vi "svl_Peak Level (1 Ch).vi"(8 "error in (no error)":errorcluster, 9 "processing state":T1(ring), 11 "scaled signal":waveform(dbl)={"t0"=timestamp(0 s since 1904-01-01), "dt"=0.0, "Y"=[]}) -> (0 "error out":errorcluster, 3 "peak level":dbl format="%.2f")   [LabVIEW 2017]
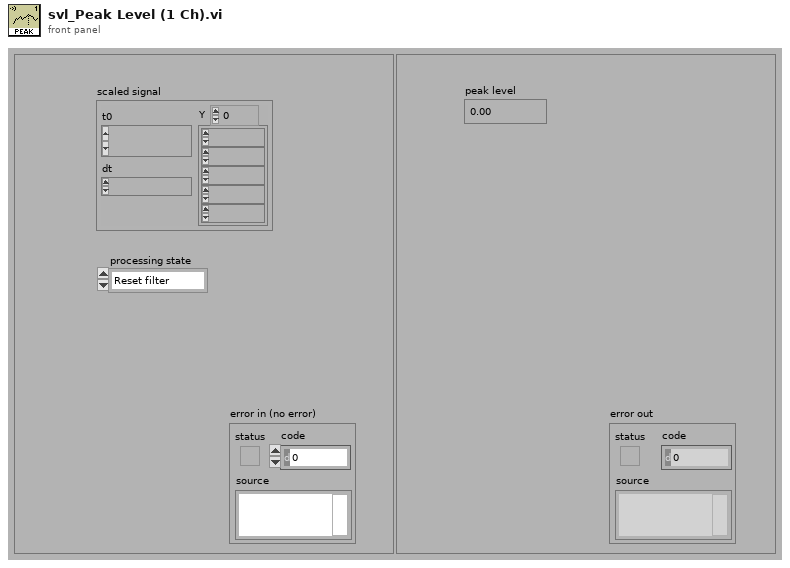
[diagram p1: front panel]
types:
  T1 = enum16{"Reset filter", "Restart averaging", "Continue processing"}
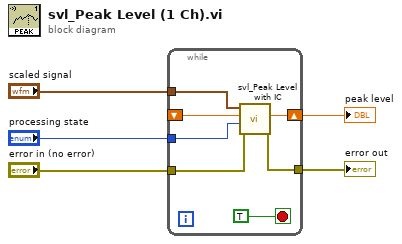
[diagram p0: block diagram]
diagram:
  n1 = while {
    shift-left: _ -> [w9]
    shift-right: [w8] -> w1
    tunnel: [w11] -> w2
    tunnel: "error in (no error)" -> [w12]
    tunnel: "processing state" -> [w7]
    tunnel: "scaled signal" -> [w6]
    stop <- TRUE stop-if-true
    n2 = call <vilib>:"svl_Peak Level with IC.vi"("error in (no error)"=w12, "processing state"=w7, "initial soundLevel"=w9, "scaled signal"=w6) -> ("error out"=w11:errorcluster, "final soundLevel"=w8:dbl)  [unwired: 6 in]
  }
  "peak level" <- w1
  "error out" <- w2
